vi "EV05全局变量1.vi"() -> ()   [LabVIEW 2013]
panel:
  out "写入超时Array":bool[](array[boolean])
  in  "波特率":u16(ring)=11 items=["250K", "500K"]
  in  "分流器型号":T1(ring)=enum."300A"
  out "退出":bool
  out "故障信息概况":string
  out "life":dbl
  out "高压校正数组":u8[](array[numeric])
  out "高压校正接收":bool
  out "CAN接收":bool
  in  "存储语言":cluster{"English":bool, "中文":bool}={"English"=TRUE, "中文"=FALSE}
  out "数据接收":bool
  out "总电压":dbl
  out "总电流":dbl
  out "单体最高电压":dbl
  out "位置1":dbl
  out "单体最低电压":dbl
  out "位置2":dbl
  out "压差":dbl
  out "SOC":dbl
  out "单体最高温度":dbl
  out "位置3":dbl
  out "单体最低温度":dbl
  out "位置4":dbl
  out "温差":dbl
  out "单体最高内阻":dbl
  out "位置5":dbl
  out "单体最低内阻":dbl
  out "位置6":dbl
  out "总内阻":dbl
  out "BMS时间":string
  out "电池故障":string
  out "电池系统故障":string
  out "硬件故障":string
  out "其他故障":string
  out "电池系统绝缘状态":string
  out "应用类型":string
  out "波特率22":string
  out "协议是否公开":string
  out "协议版本号":string
  out "SOH":dbl
  out "CAN卡类型":u32(ring)=4 items=["PCI5121"=1, "PCI9810"=2, "USBCAN1"=3, "USBCAN2"=4, "PCI9820"=5, "PCI5110"=7, "CANLite(mini)"=8, "ISA9620"=9, "ISA5420"=10, "PC104CAN"=11, "DNP9810"=13, "PCI9840B"=14, "PC104C2"=15, "PCI9820I"=16, "pec9920"=18, "USBCAN_E_U"=20, "USBCAN_2E_U"=21]
  out "CAN端口":u16(ring) items=["0", "1"]
  out "设备索引号":u16(ring) items=["0", "1", "2", "3", "4", "5", "6", "7", "8", "9", "10", "11", "12", "13", "14", "15", ""]
  out "E-U_baud":u32(ring)=393223 items=["0x060003--1000Kbps"=393219, "0x060004--800Kbps"=393220, "0x060007--500Kbps"=393223, "0x1C0008--250Kbps"=1835016, "0x1C0011--125Kbps"=1835025, "0x160023--100Kbps"=1441827, "0x1C002C--50Kbps"=1835052, "0x1600B3--20Kbps"=1441971, "0x1C00E0--10Kbps"=1835232, "0x1C01C1--5Kbps"=1835457]
  out "授权功能":bool
  out "读取超时":bool
  out "写入超时":bool
  in  "输出数组":u8[](array[numeric])
  out "流控帧 2":bool
  out "写?":bool
  out "超时":bool
  out "流控帧":bool
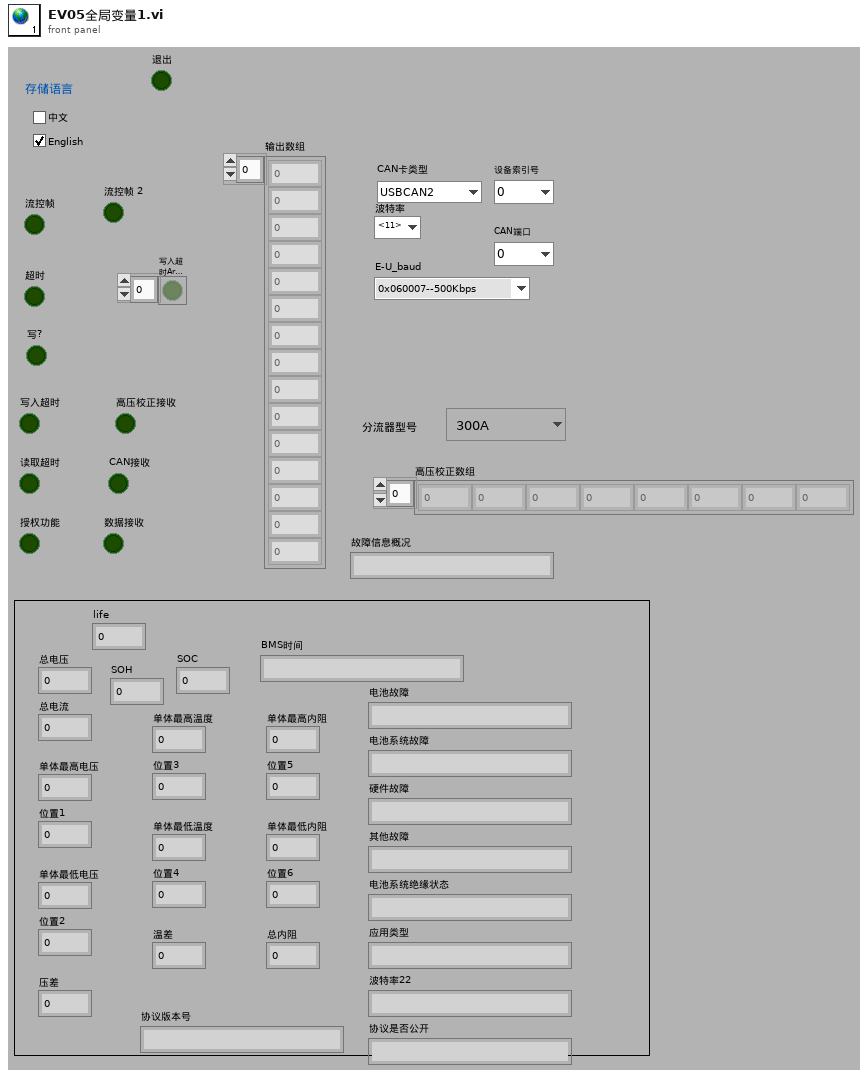
[diagram p1: front panel]
types:
  T1 = enum16{"选择分流器型号", "100A", "200A", "300A", "400A", "500A", "600A", "700A", "800A", "900A", "1000A"}
diagram:
